vi "LJUD_eTCConfig.vi"(0 "Handle In":i32, 1 "aEnableCounters":i32[](array[numeric]), 5 "aEnableTimers":i32[](array[numeric]), 7 "aTimerModes":i32[](array[numeric]), 9 "aTimerValues":dbl[](array[numeric]) format="%.2f", 11 "error in":errorcluster, 12 "TCPinOffset":i32, 13 "TimerClockBaseIndex":i32, 14 "TimerClockDivisor":i32) -> (4 "Handle Out":i32, 15 "error out":errorcluster)   [LabVIEW 2021]
doc: "This is an e-function that can configure\nand initialize all the timers and counters\nin a single call. A somewhat complex\nfunction, but can help reinforce the\ninteraction between the different timers\nand counters on the device.\n\nSee Sections 4.2 and 4.3 of the device's\ndatasheet for more information."
uses:
  labjackud.dll
panel:
  # "This is an e-function that can configure\nand initialize all the timers and counters\nin a single call.  A somewhat complex\nfunction, but can help reinforce the\ninteraction between the different timers\nand counters on the device.\n\nSee Sections 4.2 and 4.3 of the device's\ndatasheet for more information."
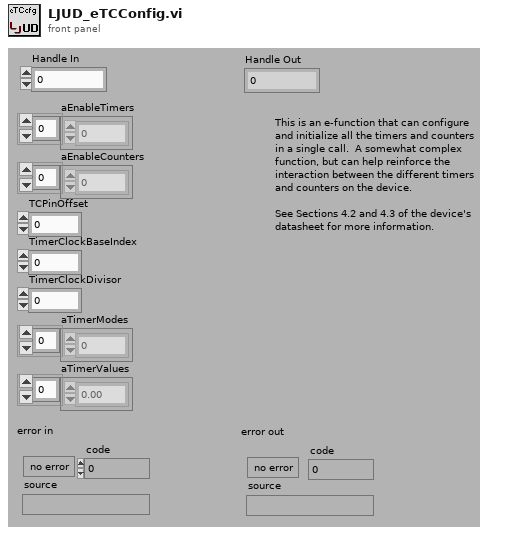
[diagram p1: front panel]
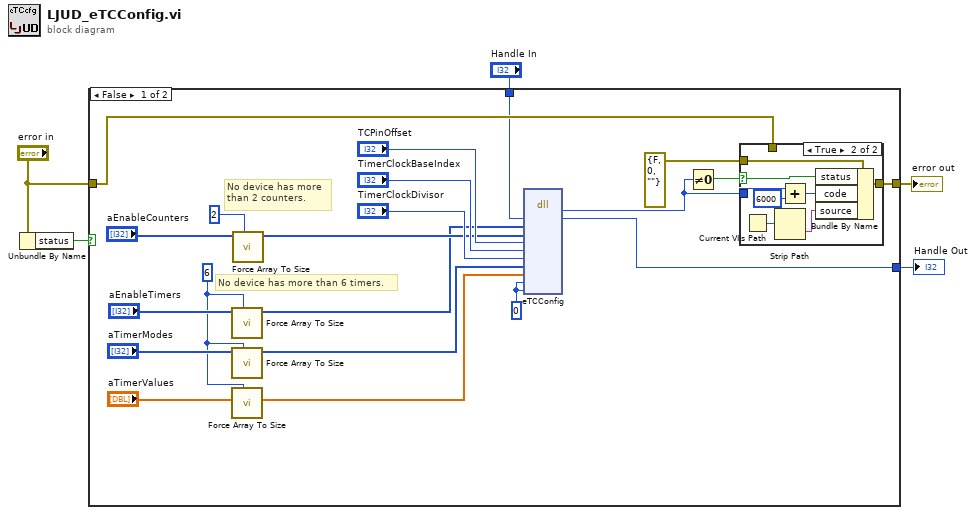
[diagram p0: block diagram]
diagram:
  n1 = Unbundle By Name("error in") -> ("status"=w4:bool)
  n2 = case shown="False" w4 {
    tunnel: [w23 w37] -> w5
    tunnel: "error in" -> [w22 w37]
    tunnel: "Handle In" -> [w7 w36]
    tunnel: [w6 w36] -> w1
    frame False {
      w8 = 6 ("# Elements")
      w18 = 0 ("GoError")
      # "No device has more than 6 timers."
      # "No device has more\nthan 2 counters."
      n3 = call "Force Array To Size.vi"("# Elements"=w8, "I32 Array In"="aEnableTimers") -> ("I32 Array Out"=w9:i32[])  [unwired: 6 in, 3 out]
      n4 = call "Force Array To Size.vi"("# Elements"=w8, "I32 Array In"="aTimerModes") -> ("I32 Array Out"=w11:i32[])  [unwired: 6 in, 3 out]
      n5 = call "Force Array To Size.vi"("# Elements"=w8, "DBL Array In"="aTimerValues") -> ("DBL Array Out"=w13:dbl[])  [unwired: 6 in, 3 out]
      n6 = call "Force Array To Size.vi"("# Elements"=2, "I32 Array In"="aEnableCounters") -> ("I32 Array Out"=w16:i32[])  [unwired: 6 in, 3 out]
      n7 = dll-call lib="labjackud.dll" fn="eTCConfig"("Handle"=w7, "aEnableTimers"=w9, "aEnableCounters"=w16, "TCPinOffset"="TCPinOffset", "TimerClockBaseIndex"="TimerClockBaseIndex", "TimerClockDivisor"="TimerClockDivisor", "aTimerModes"=w11, "aTimerValues"=w13, "Reserved1"=w18, "Reserved2"=w18) -> (w24:i32, "Handle"=w6:i32)  [unwired: 12 in, 2 out]
      n8 = Not Equal To 0?(x=w24) -> (x != 0?=w25:bool)
      n9 = case shown="True" w25 {
        selector: w25 -> [_ w34]
        tunnel: [w27 w35] -> w23
        tunnel: errorcluster {"status"=FALSE, "code"=0, "source"=""} ("error IO") -> [_ w33]
        tunnel: w24 -> [_ w29]
        tunnel: w22 -> [w27 _]
        frame False {
        }
        frame True {
          n10 = Current VI's Path() -> (path=w31:path)
          n11 = Strip Path(path=w31) -> (name=w32:string)  [unwired: 1 out]
          n12 = Add(x=w29, y=6000) -> (x+y=w30:i32)
          n13 = Bundle By Name(cluster=w33, "status"=w34, "code"=w30, "source"=w32) -> (w35:errorcluster)
        }
      }
    }
    frame True {
    }
  }
  "error out" <- w5
  "Handle Out" <- w1
